vi "SPI Engine Core 128-bit.vi"(6 "Ready for Output":bool, 9 "Input Valid":bool, 10 "SPI Information In":T1={"Start Strobe"=FALSE, "SPI Data"=[FALSE, FALSE, FALSE, FALSE, FALSE, FALSE, FALSE, FALSE, FALSE, FALSE, FALSE, FALSE, FALSE, FALSE, FALSE, FALSE, FALSE, FALSE, FALSE, FALSE, FALSE, FALSE, FALSE, FALSE, FALSE, FALSE, FALSE, FALSE, FALSE, FALSE, FALSE, FALSE, FALSE, FALSE, FALSE, FALSE, FALSE, FALSE, FALSE, FALSE, FALSE, FALSE, FALSE, FALSE, FALSE, FALSE, FALSE, FALSE, FALSE, FALSE, FALSE, FALSE, FALSE, FALSE, FALSE, FALSE, FALSE, FALSE, FALSE, FALSE, FALSE, FALSE, FALSE, FALSE, FALSE, FALSE, FALSE, FALSE, FALSE, FALSE, FALSE, FALSE, FALSE, FALSE, FALSE, FALSE, FALSE, FALSE, FALSE, FALSE, FALSE, FALSE, FALSE, FALSE, FALSE, FALSE, FALSE, FALSE, FALSE, FALSE, FALSE, FALSE, FALSE, FALSE, FALSE, FALSE, FALSE, FALSE, FALSE, FALSE, FALSE, FALSE, FALSE, FALSE, FALSE, FALSE, FALSE, FALSE, FALSE, FALSE, FALSE, FALSE, FALSE, FALSE, FALSE, FALSE, FALSE, FALSE, FALSE, FALSE, FALSE, FALSE, FALSE, FALSE, FALSE, FALSE, FALSE, FALSE], "SPI Settings"={"Chip Select ID"=0, "SPI Physical Settings"={"Divide Value"=0, "Transfer Length (bits)"=1, "CS Asserted Polarity"=FALSE, "Clock Polarity (CPOL)"=FALSE, "Clock Phase (CPHA)"=FALSE, "Lengthen MISO Setup"=FALSE, "Direction Change Bit"=0, "MOSI Starts as Output"=FALSE, "Tristatable MOSI"=FALSE}}} {"SPI Settings"."SPI Physical Settings"."Direction Change Bit" max=64 step=1; "SPI Settings"."SPI Physical Settings"."Transfer Length (bits)" min=1 max=64 step=1}, 11 "SPI DIO Input":T7) -> (1 "Output Valid":bool, 2 "SPI Output Data":T5, 3 "SPI DIO Output":T6, 4 "Ready For Input":bool, 5 "Chip Select ID":u8)   [LabVIEW 2015, in "SPI API.lvlib"]
doc: "This VI performs the actual SPI Transactions. It wraps the SPI Core with added functionality of 4-Wire Handshake"
uses:
  SPI API.lvlib
  <userlib>/_NI SPI IP/FPGA/Controllers/Public/Spi Master Inputs.ctl
  <userlib>/_NI SPI IP/FPGA/Controllers/Public/Spi Master Outputs.ctl
  Controls/SPI API Response Data 128-bit.ctl
  Controls/SPI API Data 128-bit.ctl
  Controls/SPI API Transaction Packet 128-bit.ctl
  Controls/SPI Transaction Settings.ctl
  <userlib>/_NI SPI IP/FPGA/Controllers/Public/Transfer Settings.ctl
  SPI Engine.Core.Input Buffer 128-bit.vi
  Custom SPI IP/Spi Master 128-bit.vi
  SPI Engine.Core.Output Buffer 128-bit.vi
  <userlib>/_NI SPI IP/FPGA/Controllers/NI SPI IP FPGA.lvlib
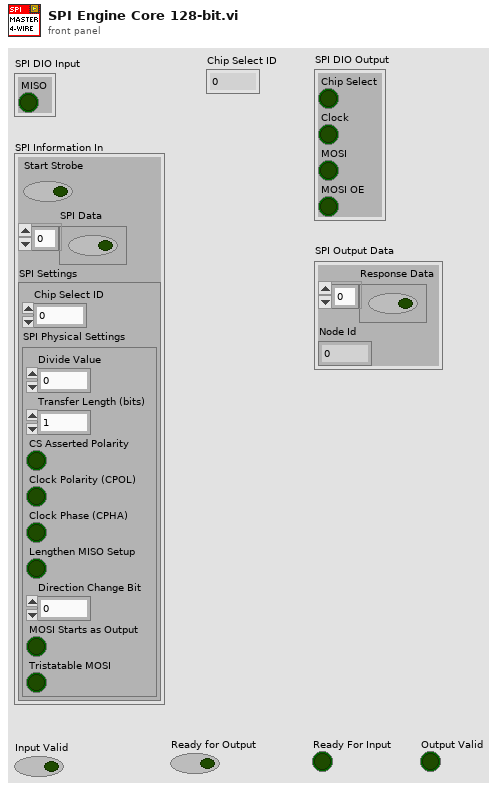
[diagram p1: front panel]
types:
  T1 = typedef "SPI API.lvlib/SPI API Transaction Packet 128-bit.ctl" = cluster{"Start Strobe":bool, "SPI Data":T2, "SPI Settings":T3}
  T2 = typedef "SPI API.lvlib/SPI API Data 128-bit.ctl" = bool[]
  T3 = typedef "SPI API.lvlib/SPI Transaction Settings.ctl" = cluster{"Chip Select ID":u8, "SPI Physical Settings":T4}
  T4 = typedef "NI SPI IP FPGA.lvlib/Transfer Settings.ctl" = cluster{"Divide Value":u8, "Transfer Length (bits)":u8, "CS Asserted Polarity":bool, "Clock Polarity (CPOL)":bool, "Clock Phase (CPHA)":bool, "Lengthen MISO Setup":bool, "Direction Change Bit":u8, "MOSI Starts as Output":bool, "Tristatable MOSI":bool}
  T5 = typedef "SPI API.lvlib/SPI API Response Data 128-bit.ctl" = cluster{"Response Data":T2, "Node Id":u16}
  T6 = typedef "NI SPI IP FPGA.lvlib/Spi Master Outputs.ctl" = cluster{"Chip Select":bool, "Clock":bool, "MOSI":bool, "MOSI OE":bool}
  T7 = typedef "NI SPI IP FPGA.lvlib/Spi Master Inputs.ctl" = cluster{"MISO":bool}
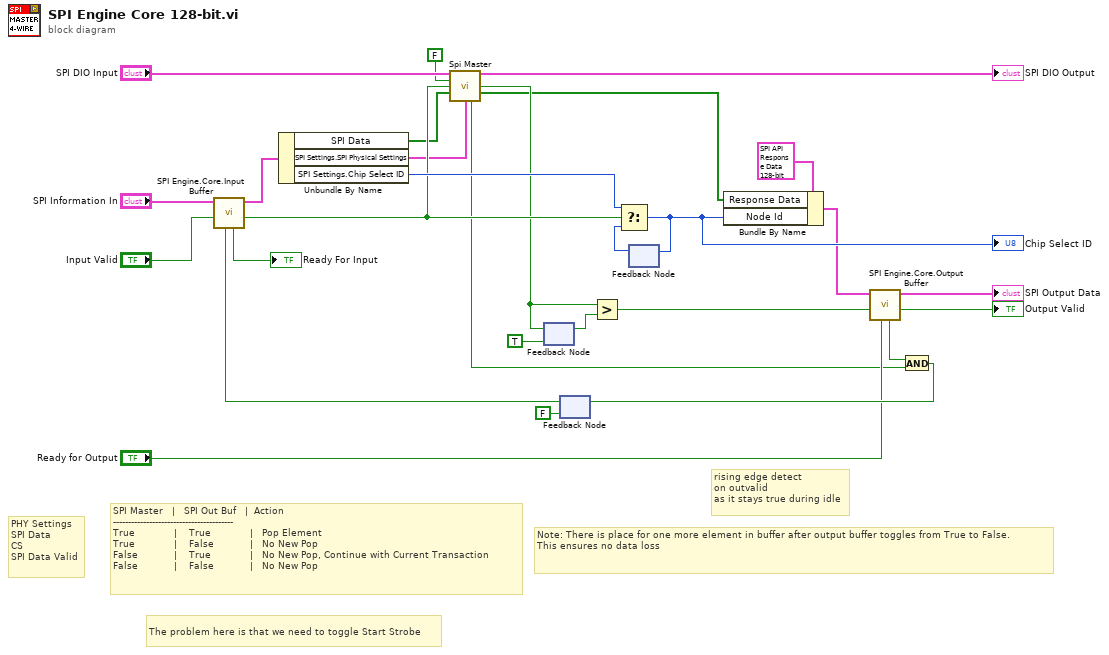
[diagram p0: block diagram]
diagram:
  # "rising edge detect\non outvalid\nas it stays true during idle"
  # "PHY Settings\nSPI Data\nCS\nSPI Data Valid"
  # "The problem here is that we need to toggle Start Strobe"
  # "Note: There is place for one more element in buffer after output buffer toggles from True to False.\nThis ensures no data loss"
  # "SPI Master   |   SPI Out Buf   |  Action\n----------------------------------------\nTrue             |    True             |   Pop Element\nTrue             |    False            |   No New Pop \nFalse            |    True             |   No New Pop, Continue with Current Transaction\nFalse            |    False            |   No New Pop"
  n1 = feedback #1(TRUE ("read data valid")) -> (w24:bool)
  n2 = feedback #2(FALSE) -> (w20:bool)
  n3 = call-poly "SPI Engine.Core.Input Buffer.vi"("Ready for Output"=w20, "Input Valid"="Input Valid", "SPI Information In"="SPI Information In") -> ("Output Valid"=w9:bool, "SPI Information Out"=w11:T1, "Ready For Input"=→"Ready For Input":bool)  [unwired: 6 in]
  n4 = Unbundle By Name(w11) -> ("SPI Data"=w8:T2, "SPI Settings.SPI Physical Settings"=w7:T4, "SPI Settings.Chip Select ID"=w22:u8)
  n5 = call-poly "Spi Master.vi"("spi input"="SPI DIO Input", "manual assert chip select"=FALSE, "start strobe"=w9, "data to write"=w8, "spi transfer settings"=w7) -> ("spi output"=→"SPI DIO Output":T6, "read data valid"=w4:bool, "read data"=w3:bool[], "ready for input"=w6:bool)  [unwired: 7 in]
  n6 = feedback-in #1(w4) -> ()
  n7 = Greater?(x=w4, y=w24) -> (0:w16:bool)
  n8 = feedback #3() -> (w25:u8)  [unwired: 1 in]
  n9 = Select(t=w22, s=w9, f=w25) -> (s? t:f=w23:u8)
  "Chip Select ID" <- w23
  n10 = feedback-in #3(w23) -> ()
  n11 = Bundle By Name(cluster=T5 {"Response Data"=[FALSE, FALSE, FALSE, FALSE, FALSE, FALSE, FALSE, FALSE, FALSE, FALSE, FALSE, FALSE, FALSE, FALSE, FALSE, FALSE, FALSE, FALSE, FALSE, FALSE, FALSE, FALSE, FALSE, FALSE, FALSE, FALSE, FALSE, FALSE, FALSE, FALSE, FALSE, FALSE, FALSE, FALSE, FALSE, FALSE, FALSE, FALSE, FALSE, FALSE, FALSE, FALSE, FALSE, FALSE, FALSE, FALSE, FALSE, FALSE, FALSE, FALSE, FALSE, FALSE, FALSE, FALSE, FALSE, FALSE, FALSE, FALSE, FALSE, FALSE, FALSE, FALSE, FALSE, FALSE, FALSE, FALSE, FALSE, FALSE, FALSE, FALSE, FALSE, FALSE, FALSE, FALSE, FALSE, FALSE, FALSE, FALSE, FALSE, FALSE, FALSE, FALSE, FALSE, FALSE, FALSE, FALSE, FALSE, FALSE, FALSE, FALSE, FALSE, FALSE, FALSE, FALSE, FALSE, FALSE, FALSE, FALSE, FALSE, FALSE, FALSE, FALSE, FALSE, FALSE, FALSE, FALSE, FALSE, FALSE, FALSE, FALSE, FALSE, FALSE, FALSE, FALSE, FALSE, FALSE, FALSE, FALSE, FALSE, FALSE, FALSE, FALSE, FALSE, FALSE, FALSE, FALSE, FALSE, FALSE], "Node Id"=0} ("SPI Response"), "Response Data"=w3, "Node Id"=w23) -> (w18:T5)
  n12 = call-poly "SPI Engine.Core.Output Buffer.vi"("Ready for Output"="Ready for Output", "Input Valid"=w16, "Input Data"=w18) -> ("Output Valid"=→"Output Valid":bool, "Output Data"=→"SPI Output Data":T5, "Ready For Input"=w13:bool)  [unwired: 6 in]
  n13 = And(x=w13, y=w6) -> (x .and. y?=w28:bool)
  n14 = feedback-in #2(w28) -> ()
